vi "Get Type Name.vi"(11 "PS in":refnum<class "Power Supply.lvclass">) -> (2 "Type Name":string)   [LabVIEW 2019, in "Power Supply.lvlib" / "Power Supply.lvclass"]
uses:
  Power Supply.lvclass
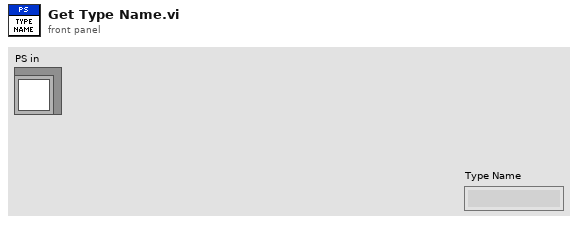
[diagram p1: front panel]
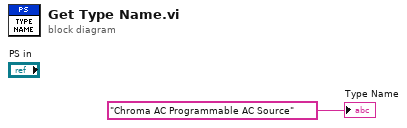
[diagram p0: block diagram]
diagram:
  "Type Name" <- "Chroma AC Programmable AC Source" ("Type Name")
